vi "Convert_Styx2Register.vi"(6 "1299R?":bool caption="1299R? (F)", 8 "Styx File Tags - Enum":variant) -> (0 "String":string)   [LabVIEW 2010]
doc: "This VI converts the Styx enum tag to the register name (from datasheet) for usage in the process of the controls.\n\nInput:\nStyx File Tags - Enum -> styx enum to convert to register name\n\nOutput:\nString -> register name"
uses:
  Estyx/TYP_ADS1299Estyx File Enum.ctl
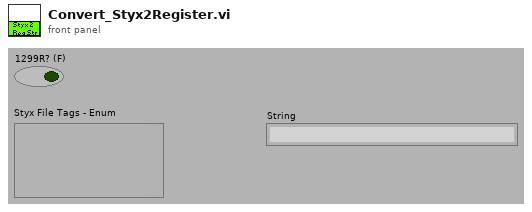
[diagram p1: front panel]
types:
  T1 = typedef "TYP_ADS1299Estyx File Enum.ctl" = enum16{"|version", "|id", "ads1299evm|blocksize_samples", "ads1299evm|acquire", "ads1299evm|data", "conf|ch1set", "conf|ch2set", "conf|ch3set", "conf|ch4set", "conf|ch5set", "conf|ch6set", "conf|ch7set", "conf|ch8set", "conf|config1", "conf|config2", "conf|config3", "conf|devid", "conf|gpio", "conf|loff", "conf|loffflip", "conf|loffsensn", "conf|loffsensp", "conf|loffstatn", "conf|loffstatp", "conf|misc2", "conf|misc1", "conf|biassensn", "conf|biassensp", "conf|reset", "conf|sleep", "conf|config4", "led|dp", "led|seg", "led|ch", "mmb0|pll", "mmb0|clkout", "mmb0|clkfreq"}
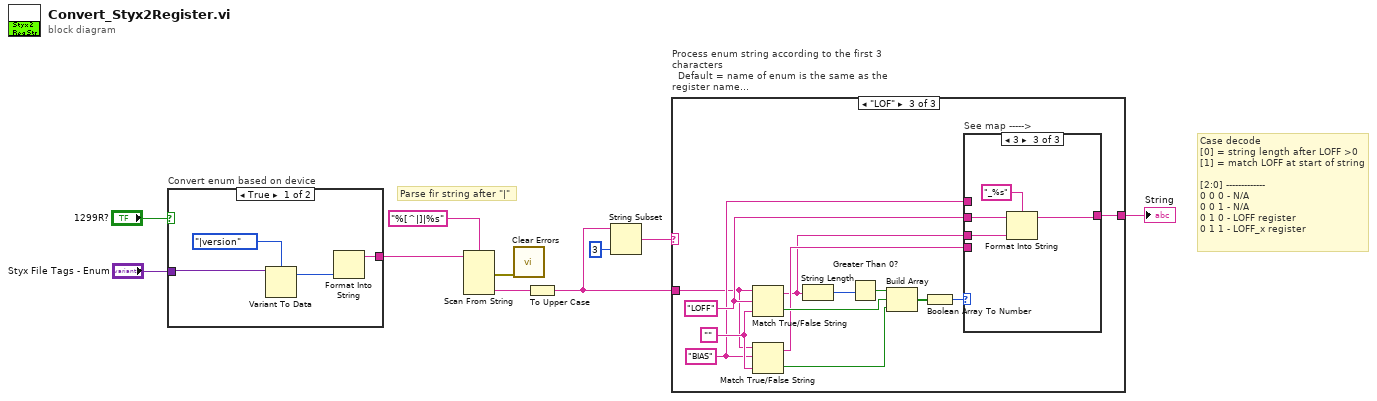
[diagram p0: block diagram]
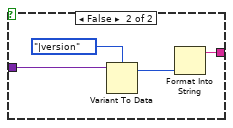
[diagram p2: hidden frame]
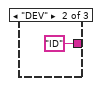
[diagram p4: hidden frame]
diagram:
  # "Parse fir string after \"|\""
  # "Case decode\n[0] = string length after LOFF >0\n[1] = match LOFF at start of string\n\n[2:0] -------------\n0 0 0 - N/A\n0 0 1 - N/A\n0 1 0 - LOFF register\n0 1 1 - LOFF_x register"
  n1 = case "Convert enum based on device" shown="True" "1299R?" {
    tunnel: [w14 w18] -> w10
    tunnel: "Styx File Tags - Enum" -> [w12 w16]
    frame True {
      n2 = Variant To Data(Variant=w12, type=TYP_ADS1299Estyx_File_Enum."|version" ("Styx File Tags - Enum")) -> (data=w13:T1)  [unwired: 1 in, 1 out]
      n3 = Format Into String(w13) -> (resulting string=w14:string)  [unwired: 3 in, 1 out]
    }
    frame False {
      n4 = Variant To Data(Variant=w16, type=TYP_ADS1299Estyx_File_Enum."|version" ("Styx File Tags - Enum")) -> (data=w17:T1)  [unwired: 1 in, 1 out]
      n5 = Format Into String(w17) -> (resulting string=w18:string)  [unwired: 3 in, 1 out]
    }
  }
  n6 = Scan From String(format string="%[^|]|%s", input string=w10) -> (error out=w6:errorcluster, output 2=w8:string)  [unwired: 2 in, 5 out]
  n7 = call <vilib>:"Clear Errors.vi"("error in (no error)"=w6) -> ()  [unwired: 7 out]
  n8 = To Upper Case(1:w8) -> (0:w4:string)
  n9 = String Subset(string=w4, length (rest)=3 ("length (rest)")) -> (substring=w5:string)  [unwired: 1 out]
  n10 = case "Process enum string according to the first 3 characters\n  Default = name of enum is the same as the register name\n  DEV = output \"ID\" for the register name\n  LOF or BIAS = add/insert \"_\" to create register name" shown="\"LOF\"" w5 {
    tunnel: [w19 "ID" w32] -> w7
    tunnel: w4 -> [w19 _ w22]
    frame Default {
    }
    frame "DEV" {
    }
    frame "LOF" {
      w24 = "BIAS" ("true string")
      w26 = ""
      w27 = "LOFF" ("true string")
      n11 = Match True/False String(2:w26, 3:w27, 4:w22) -> (0:w30:bool, 1:w21:string)
      n12 = Match True/False String(2:w26, 3:w24, 4:w22) -> (0:w25:bool, 1:w23:string)
      n13 = String Length(string=w21) -> (length=w33:i32)
      n14 = Greater Than 0?(x=w33) -> (x > 0?=w31:bool)
      n15 = Build Array(w31, w30, w25) -> (w28:bool[])
      n16 = Boolean Array To Number(Boolean array=w28) -> (number=w29:u32)
      n17 = case "See map ----->" shown="3" w29 {
        tunnel: w27 -> [_ w35 w39]
        tunnel: w21 -> [w34 _ w38]
        tunnel: [w34 w35 w36] -> w32
        tunnel: w24 -> [_ _ _]
        tunnel: w23 -> [_ _ _]
        frame Default {
        }
        frame 2 {
        }
        frame 3 {
          n18 = Format Into String(format string="_%s", initial string=w39, w38) -> (resulting string=w36:string)  [unwired: 1 in, 1 out]
        }
      }
    }
  }
  "String" <- w7
